vi "Get DI Settings from DI TaskName in Dict.vi"(8 "error in (no error)":errorcluster, 10 "DI TaskName":string, 11 "DAQ":refnum<class "DAQ.lvclass">) -> (0 "error out":errorcluster, 2 "DI Settings":T1, 3 "DAQ":refnum<class "DAQ.lvclass">)   [LabVIEW 2017, in "DAQ.lvclass"]
doc: "Developed by Kevin Thompson\nkevin@thompsonengineering.net\n\nCopyright 2018-2020\nThompson Engineering, LLC"
uses:
  DAQ.lvclass
  DataTypes/TD DI Instrument Settings--cluster.ctl
  DAQ.lvclass/DAQ.ctl
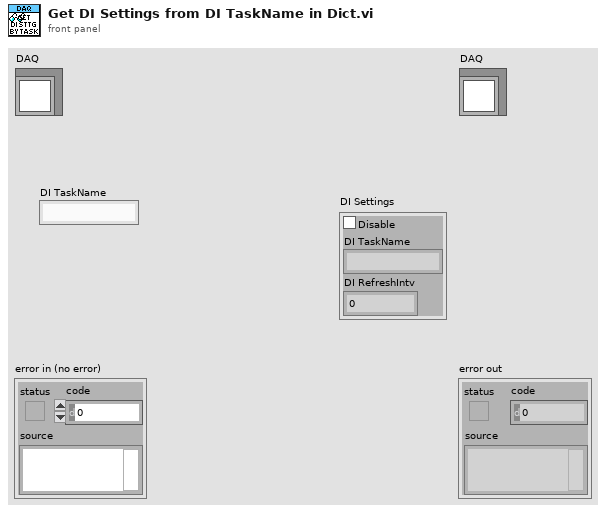
[diagram p1: front panel]
types:
  T1 = typedef "DAQ.lvclass/TD DI Instrument Settings--cluster.ctl" = cluster{"Disable":bool, "DI TaskName":string, "DI RefreshIntv":i32}
  T2 = typedef "TD Dynamic CVT DVR--ref.ctl" = refnum<data-value>
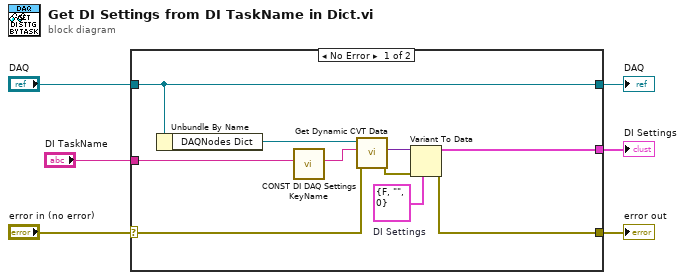
[diagram p0: block diagram]
diagram:
  n1 = case shown="No Error" "error in (no error)" {
    selector: "error in (no error)" -> [w14 w17]
    tunnel: [w13 w17] -> w5
    tunnel: [w16 w18] -> w3
    tunnel: "DAQ" -> [w16 w18]
    tunnel: "DI TaskName" -> [w8 _]
    tunnel: [w10 _] -> w1
    frame No Error {
      w9 = T1 {"Disable"=FALSE, "DI TaskName"="", "DI RefreshIntv"=0}  # DI Settings
      n2 = Unbundle By Name(w16) -> ("DAQNodes Dict"=w15:T2)
      n3 = call "CONST DI DAQ Settings KeyName.vi"("DI TaskName"=w8) -> ("DI DAQ Settings (KeyName)"=w7:string)  [unwired: 10 in]
      n4 = call <vilib>:"Get Dynamic CVT Data.vi"("error in (no error)"=w14, "DataName"=w7, "dCVT DVR"=w15) -> ("error out"=w12:errorcluster, "value"=w11:variant)  [unwired: 5 in, 2 out]
      n5 = Variant To Data(error in=w12, type=w9, Variant=w11) -> (data=w10:T1, error out=w13:errorcluster)
    }
    frame Error {
    }
  }
  "error out" <- w5
  "DAQ" <- w3
  "DI Settings" <- w1
